vi "Page_Routing_Templates_ReadShared.vi"(6 "ctl references":T1, 7 "MethodVI names":string[](array[string]), 8 "error in (no error)":errorcluster, 11 "AB_RESTfulWebService in":refnum<class "AB_RESTfulWebService.lvclass">) -> (0 "error out":errorcluster, 3 "AB_RESTfulWebService out":refnum<class "AB_RESTfulWebService.lvclass">)   [LabVIEW 2020, in "AB_RESTfulWebService.lvclass"]
uses:
  <vilib>/AppBuilder/AB_Classes/RESTful/AB_RESTfulWebService.lvclass
  <resource>/Framework/Providers/Builds/AppBuilder/AB_UI_Page_Routing_Templates_References.ctl
  <vilib>/AppBuilder/AB_Classes/RESTful/AB_RESTfulWebService.lvclass/AB_RESTfulWebService.ctl
  <vilib>/Utility/miscctls.llb/LVRowAndColumnUnsignedTypeDef.ctl
  <vilib>/Utility/miscctls.llb/LVRowAndColumnTypeDef.ctl
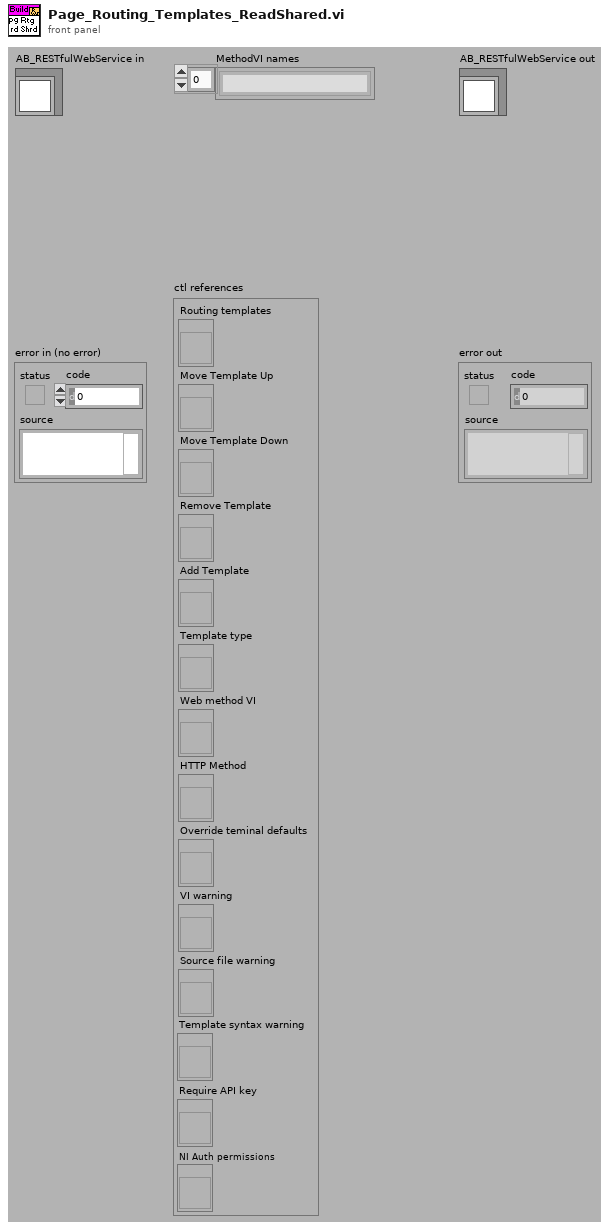
[diagram p1: front panel]
types:
  T1 = typedef "AB_UI_Page_Routing_Templates_References.ctl" = cluster{"Routing templates":refnum<vi>, "Move Template Up":refnum<vi>, "Move Template Down":refnum<vi>, "Remove Template":refnum<vi>, "Add Template":refnum<vi>, "Template type":refnum<vi>, "Web method VI":refnum<vi>, "HTTP Method":refnum<vi>, "Override teminal defaults":refnum<vi>, "VI warning":refnum<vi>, "Source file warning":refnum<vi>, "Template syntax warning":refnum<vi>, "Require API key":refnum<vi>, "NI Auth permissions":refnum<vi>}
  T2 = typedef "LVRowAndColumnUnsignedTypeDef.ctl" = cluster{"Row":u32, "Column":u32}
  T3 = typedef "LVRowAndColumnTypeDef.ctl" = cluster{"Row":i32, "Column":i32}
  T4 = typedef "AB_RESTful_RoutingTemplate.ctl" = cluster{"Template":string, "Routing Type":T5, "HTTP Method Type":T6, "VIName":string, "Default String":string, "Require API key":bool, "Auth permissions":string[], "eng_Static Alias":string, "Required Privilege":string}
  T5 = typedef "AB_RESTful_RoutingType.ctl" = enum32{"Method", "Static"}
  T6 = typedef "AB_RESTful_HTTPMethodType.ctl" = enum32{"GET", "POST", "PUT", "DELETE"}
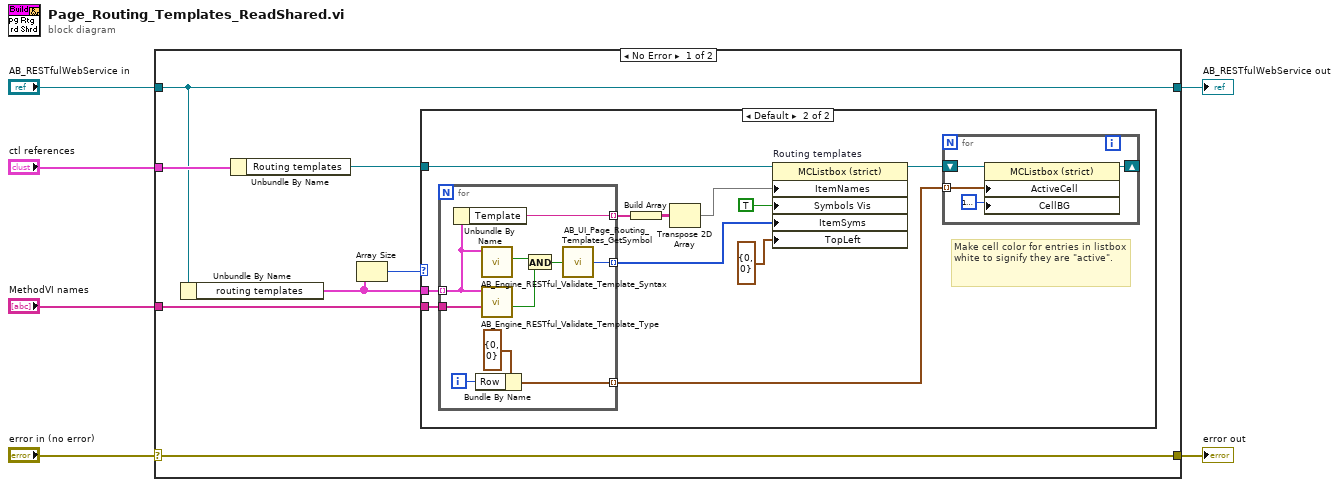
[diagram p0: block diagram]
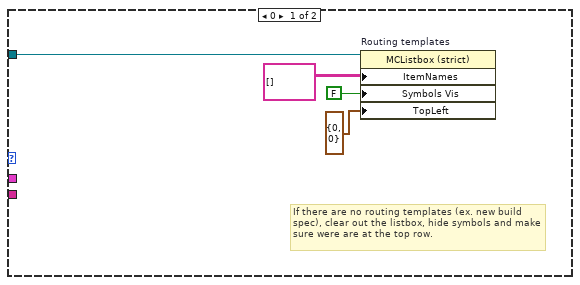
[diagram p2: hidden frame]
diagram:
  n1 = case shown="No Error" "error in (no error)" {
    selector: "error in (no error)" -> [w13 w44]
    tunnel: [w13 w44] -> w5
    tunnel: [w9 w43] -> w3
    tunnel: "AB_RESTfulWebService in" -> [w9 w43]
    tunnel: "ctl references" -> [w12 _]
    tunnel: "MethodVI names" -> [w8 _]
    frame No Error {
      n2 = Unbundle By Name(w9) -> ("routing templates"=w10:T4[])
      n3 = Unbundle By Name(w12) -> ("Routing templates"=w7:refnum<vi>)
      n4 = Array Size(array=w10) -> (size(s)=w11:i32)
      n5 = case shown="Default" w11 {
        tunnel: w10 -> [_ w26]
        tunnel: w8 -> [_ w21]
        tunnel: w7 -> [w17 w25]
        frame 0 {
          # "If there are no routing templates (ex. new build spec), clear out the listbox, hide symbols and make sure were are at the top row."
          n6 = property on="Routing templates" class="MCListbox (strict)"(reference=w17, "ItemNames"=string[][] [] ("Item Names"), "Symbols Vis"=FALSE ("Visible Items:Symbols Visible"), "TopLeft"=T2 {"Row"=0, "Column"=0} ("Top Left Visible Cell")) -> ()  [unwired: 1 in, 2 out]
        }
        frame Default {
          # "Make cell color for entries in listbox white to signify they are \"active\"."
          n7 = for {
            tunnel: w26 -> [w36] mode=indexing
            tunnel: [w39] -> w28 mode=indexing
            tunnel: [w40] -> w22 mode=indexing
            tunnel: w21 -> [w38]
            tunnel: [w37] -> w20 mode=indexing
            i -> [w41]
            n8 = Unbundle By Name(w36) -> ("Template"=w39:string)
            n9 = Bundle By Name(cluster=T3 {"Row"=0, "Column"=0} ("Active Cell:Active Cell"), "Row"=w41) -> (w40:T3)
            n10 = call <vilib>:"AB_Engine_RESTful_Validate_Template_Syntax.vi"("RESTful VI routing template in"=w36) -> ("valid syntax"=w33:bool)  [unwired: 10 out]
            n11 = call <vilib>:"AB_Engine_RESTful_Validate_Template_Type.vi"("source file names"=w38, "RESTful VI routing template in"=w36) -> ("template type vald"=w35:bool)  [unwired: 9 out]
            n12 = And(x=w33, y=w35) -> (x .and. y?=w34:bool)
            n13 = call <resource>:"AB_UI_Page_Routing_Templates_GetSymbol.vi"("template type vald"=w34) -> ("symbol"=w37:i32)  [unwired: 4 out]
          }
          n14 = Build Array(w28) -> (w27:string[][])
          n15 = Transpose 2D Array(2D array=w27) -> (transposed array=w24:string[][])
          n16 = property on="Routing templates" class="MCListbox (strict)"(reference=w25, "ItemNames"=w24, "Symbols Vis"=TRUE ("Visible Items:Symbols Visible"), "ItemSyms"=w20, "TopLeft"=T2 {"Row"=0, "Column"=0} ("Top Left Visible Cell")) -> (reference out=w23:refnum<vi>)  [unwired: 1 in, 1 out]
          n17 = for {
            shift-right: [w31] -> _
            shift-left: w23 -> [w32]
            tunnel: w22 -> [w30] mode=indexing
            n18 = property on="Routing templates" class="MCListbox (strict)"(reference=w32, "ActiveCell"=w30, "CellBG"=u32 16777226) -> (reference out=w31:refnum<vi>)  [unwired: 1 in, 1 out]
          }
        }
      }
    }
    frame Error {
    }
  }
  "error out" <- w5
  "AB_RESTfulWebService out" <- w3
